vi "Set Epsilon Current.vi"(10 "epsilon current":dbl, 11 "AnytimeDStar in":refnum<class "NI_Robotics_AnytimeDStar.lvclass">) -> (3 "AnytimeDStar out":refnum<class "NI_Robotics_AnytimeDStar.lvclass">)   [LabVIEW 2017, in "NI_Robotics_AnytimeDStar.lvclass"]
uses:
  <vilib>/robotics/Navigation/Anytime D Star/NI_Robotics_AnytimeDStar.lvclass
  <vilib>/robotics/Navigation/Anytime D Star/NI_Robotics_AnytimeDStar.lvclass/NI_Robotics_AnytimeDStar.ctl
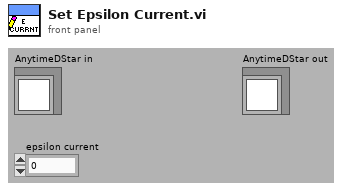
[diagram p1: front panel]
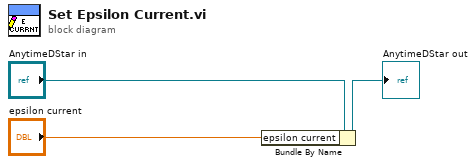
[diagram p0: block diagram]
diagram:
  n1 = Bundle By Name(cluster="AnytimeDStar in", "epsilon current"="epsilon current") -> (→"AnytimeDStar out":refnum<class "NI_Robotics_AnytimeDStar.lvclass">)
